vi "Get Plugin Name.vi"(8 "error in (no error)":errorcluster, 11 "Time Protocol in":refnum<class "Time Protocol.lvclass">) -> (0 "error out":errorcluster, 2 "String":string, 3 "Time Protocol out":refnum<class "Time Protocol.lvclass">)   [LabVIEW 2013, in "Time Protocol Actor.lvlib" / "Time Protocol.lvclass"]
uses:
  Time Protocol.lvclass
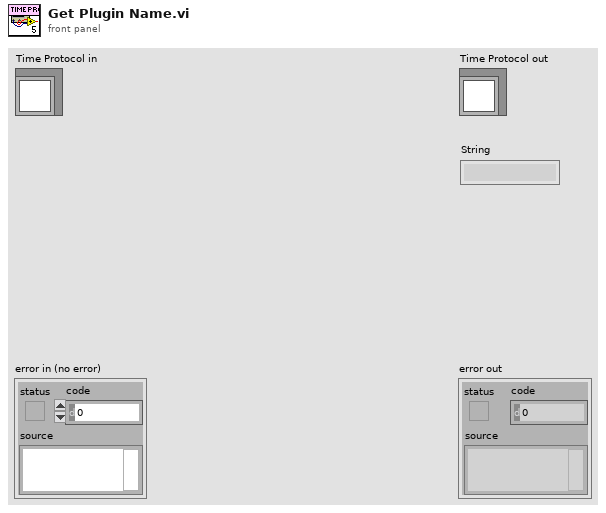
[diagram p1: front panel]
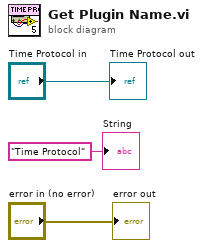
[diagram p0: block diagram]
diagram:
  "error out" <- "error in (no error)"
  "Time Protocol out" <- "Time Protocol in"
  "String" <- "Time Protocol" ("String")
